vi "Build HVAC System Directory Path.vi"(11 "Top Level Path":path) -> (3 "HAVC System Directory Path":path)   [LabVIEW 2013, in "File IO.lvlib"]
uses:
  File IO.lvlib
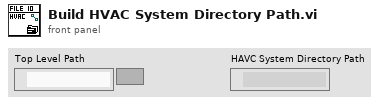
[diagram p1: front panel]
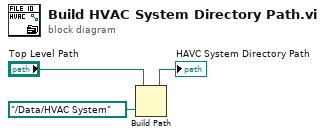
[diagram p0: block diagram]
diagram:
  n1 = Build Path(base path="Top Level Path", name or relative path=path "../Data/HVAC System") -> (appended path=→"HAVC System Directory Path":path)
